vi "HXG2_CompressorLimits.vi"(8 "error in (no error)":errorcluster, 10 "Analog In":T1, 11 "Digital In":T2) -> (0 "error out":errorcluster, 3 "Comp Contactor ON?":bool)   [LabVIEW 2012]
doc: "This VI will decide if the compressor should run based on EMO, Disch Pressure, Current Over limit and Suction Pressure limits. Output is a boolean to Compressor Contactor."
uses:
  Controls/HXG2_DigitalIn.ctl
  Controls/HXG2_AnalogIn.ctl
  Modules/CompressorContactor/HXG2comp.ctl
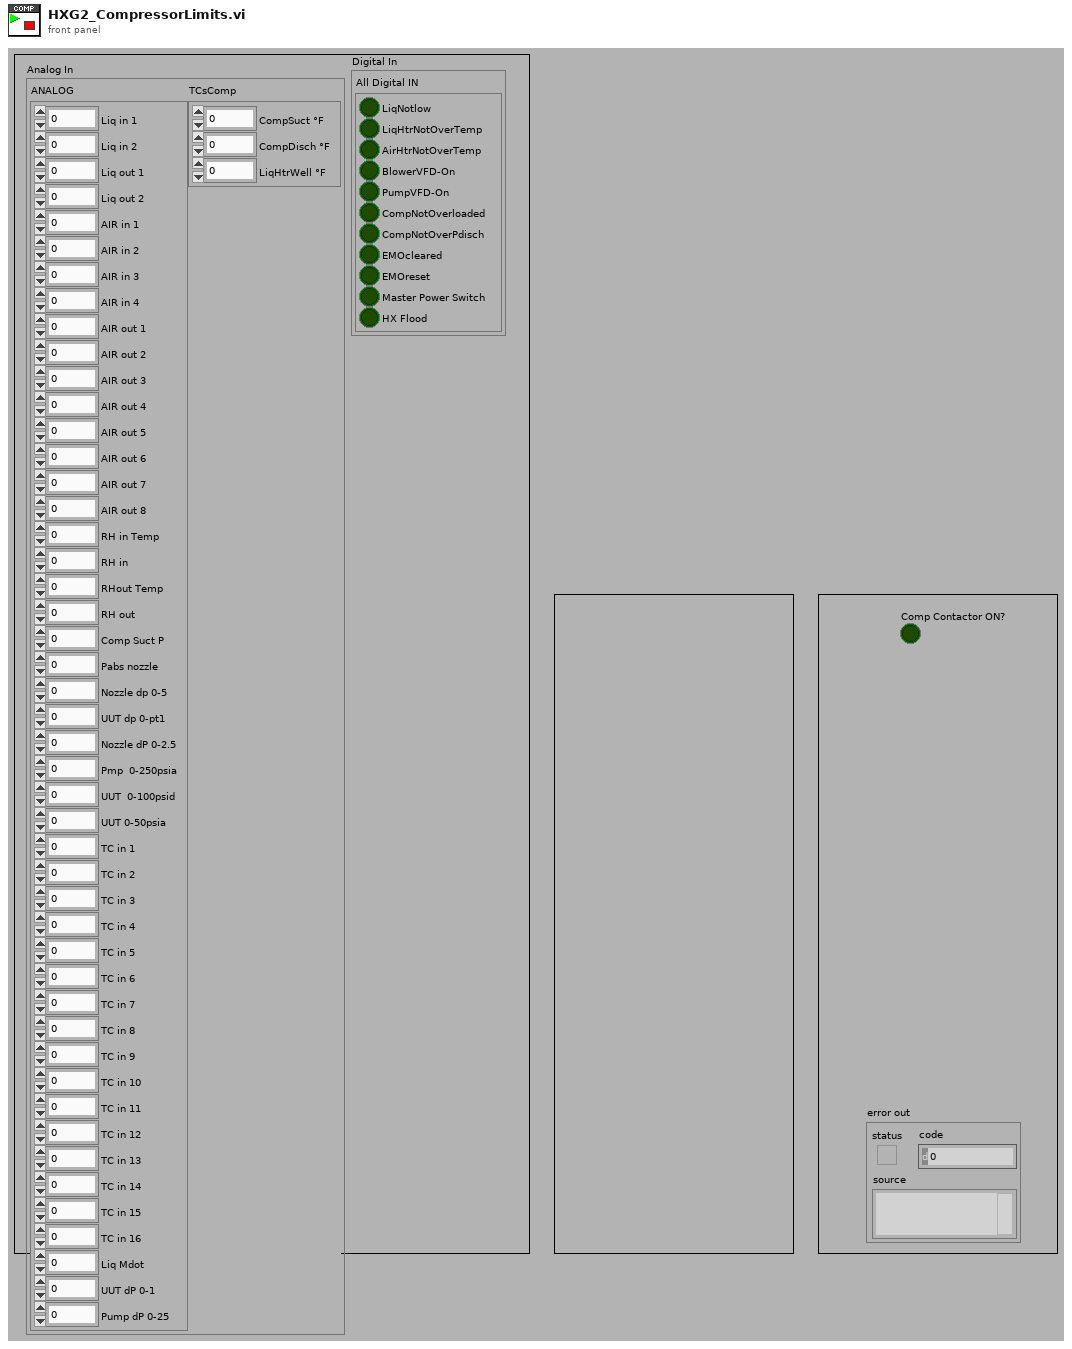
[diagram p1: front panel]
types:
  T1 = typedef "HXG2_AnalogIn.ctl" = cluster{"ANALOG":cluster{"Liq in 1":dbl, "Liq in 2":dbl, "Liq out 1":dbl, "Liq out 2":dbl, "AIR in 1":dbl, "AIR in 2":dbl, "AIR in 3":dbl, "AIR in 4":dbl, "AIR out 1":dbl, "AIR out 2":dbl, "AIR out 3":dbl, "AIR out 4":dbl, "AIR out 5":dbl, "AIR out 6":dbl, "AIR out 7":dbl, "AIR out 8":dbl, "RH in Temp":dbl, "RH in":dbl, "RHout Temp":dbl, "RH out":dbl, "Comp Suct P":dbl, "Pabs nozzle":dbl, "Nozzle dp 0-5":dbl, "UUT dp 0-pt1":dbl, "Nozzle dP 0-2.5":dbl, "Pmp  0-250psia":dbl, "UUT  0-100psid":dbl, "UUT 0-50psia":dbl, "TC in 1":dbl, "TC in 2":dbl, "TC in 3":dbl, "TC in 4":dbl, "TC in 5":dbl, "TC in 6":dbl, "TC in 7":dbl, "TC in 8":dbl, "TC in 9":dbl, "TC in 10":dbl, "TC in 11":dbl, "TC in 12":dbl, "TC in 13":dbl, "TC in 14":dbl, "TC in 15":dbl, "TC in 16":dbl, "Liq Mdot":dbl, "UUT dP 0-1":dbl, "Pump dP 0-25":dbl}, "TCsComp":cluster{"CompSuct °F  ":dbl, "CompDisch °F":dbl, "LiqHtrWell °F":dbl}}
  T2 = typedef "HXG2_DigitalIn.ctl" = cluster{"All Digital IN":cluster{"LiqNotlow":bool, "LiqHtrNotOverTemp":bool, "AirHtrNotOverTemp":bool, "BlowerVFD-On":bool, "PumpVFD-On":bool, "CompNotOverloaded":bool, "CompNotOverPdisch":bool, "EMOcleared":bool, "EMOreset":bool, "Master Power Switch":bool, "HX Flood":bool}}
  T3 = typedef "HXG2comp.ctl" = enum16{"Write", "Pass"}
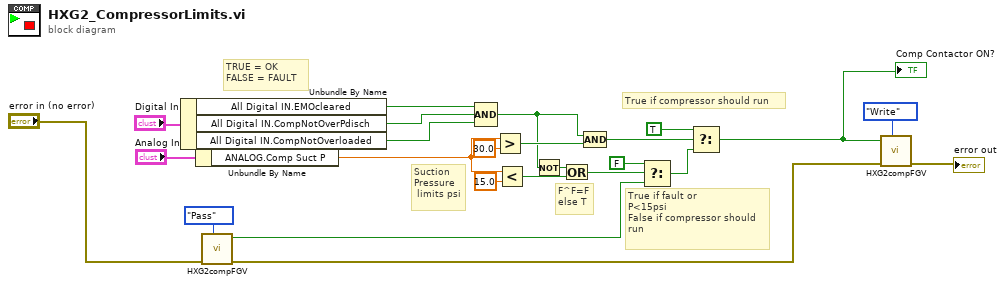
[diagram p0: block diagram]
diagram:
  # "True if compressor should run"
  # "True if fault or\nP<15psi\nFalse if compressor should\nrun"
  # "F^F=F\nelse T"
  # "TRUE = OK\nFALSE = FAULT"
  # "Suction\nPressure\n limits psi"
  n1 = Unbundle By Name("Digital In") -> ("All Digital IN.EMOcleared"=w9:bool, "All Digital IN.CompNotOverPdisch"=w8:bool, "All Digital IN.CompNotOverloaded"=w7:bool)
  n2 = Unbundle By Name("Analog In") -> ("ANALOG.Comp Suct P"=w4:dbl)
  n3 = call "HXG2compFGV.vi"("CompFGV"=HXG2comp."Pass", "error in (no error)"="error in (no error)") -> ("error out"=w3:errorcluster, "RUN?"=w6:bool)  [unwired: 8 in]
  n4 = Compound Arithmetic op=AND(w9, w8, w7) -> (w20:bool)
  n5 = Greater?(x=w4, y=30.0) -> (0:w21:bool)
  n6 = Less?(x=w4, y=15.0) -> (x < y?=w12:bool)
  n7 = Not(x=w20) -> (.not. x?=w19:bool)
  n8 = Or(x=w19, y=w12) -> (x .or. y?=w16:bool)
  n9 = Compound Arithmetic op=AND(w20, w21) -> (w18:bool)
  n10 = Select(t=FALSE ("Compressor"), s=w16, f=w6) -> (s? t:f=w14:bool)
  n11 = Select(t=TRUE ("Compressor"), s=w18, f=w14) -> (s? t:f=w2:bool)
  "Comp Contactor ON?" <- w2
  n12 = call "HXG2compFGV.vi"("CompFGV"=HXG2comp."Write", "error in (no error)"=w3, "RUN?"=w2) -> ("error out"=→"error out":errorcluster)  [unwired: 7 in, 1 out]
